vi "Write ITX (XY).vi"(4 "Commands":string, 6 "Notes":string, 8 "error in":errorcluster, 9 "wavenames":string[](array[string]), 10 "XY Array":cluster{"X  array":dbl[], "Y  Array":dbl[]}[](array[cluster]), 11 "filename":path) -> (0 "error out":errorcluster, 3 "file":path)   [LabVIEW 2016, in "Data.ITX.lvclass"]
uses:
  Data.ITX.lvclass
panel:
  out "String":string
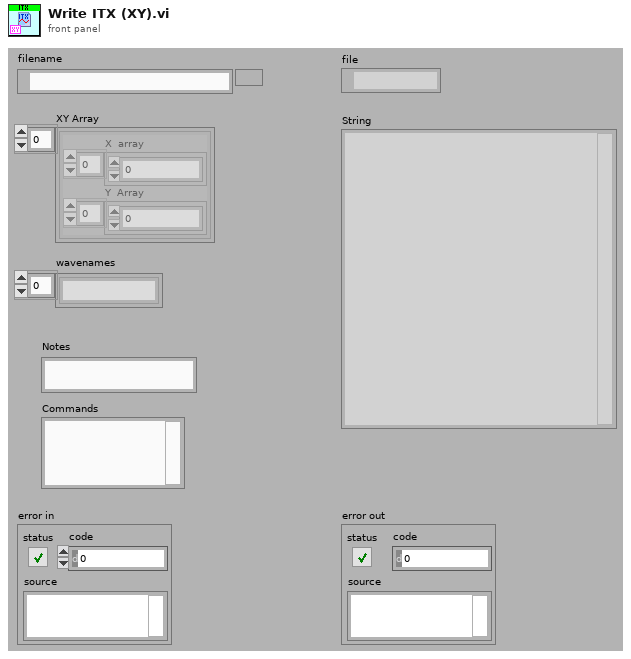
[diagram p1: front panel]
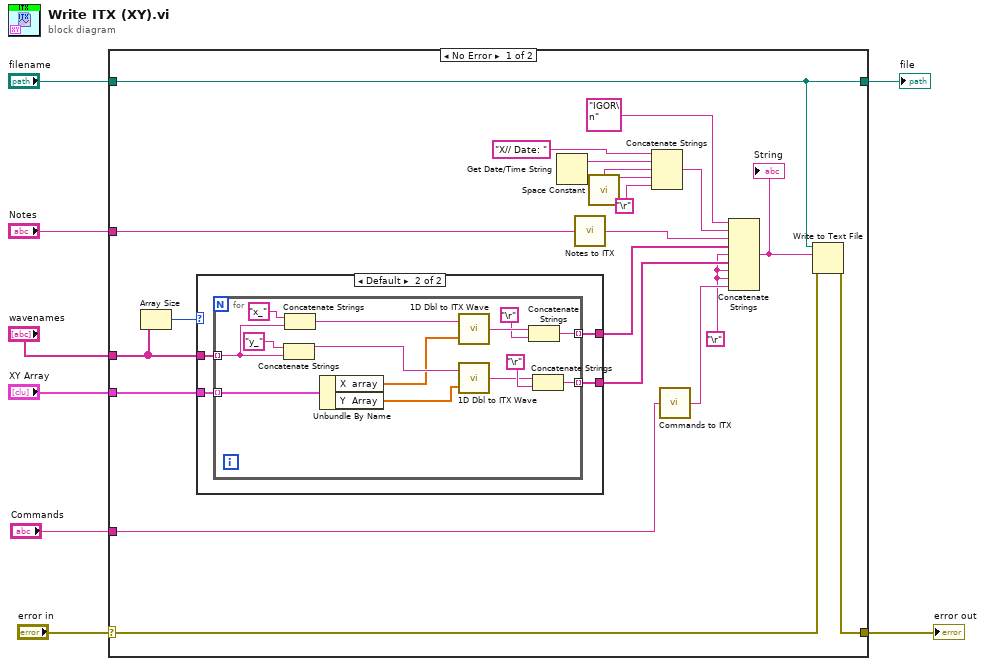
[diagram p0: block diagram]
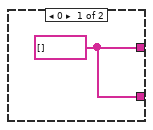
[diagram p2: hidden frame]
diagram:
  n1 = case shown="No Error" "error in" {
    selector: "error in" -> [w12 w50]
    tunnel: "filename" -> [w13 w49]
    tunnel: "wavenames" -> [w22 _]
    tunnel: "Notes" -> [w20 _]
    tunnel: "XY Array" -> [w19 _]
    tunnel: [w14 w50] -> w4
    tunnel: [w13 w49] -> w2
    tunnel: "Commands" -> [w10 _]
    frame No Error {
      w9 = "\r"
      n2 = Array Size(array=w22) -> (size(s)=w21:i32)
      n3 = case shown="Default" w21 {
        tunnel: w22 -> [_ w34]
        tunnel: w19 -> [_ w33]
        tunnel: [w30 w32] -> w24
        tunnel: [w30 w31] -> w11
        frame 0 {
          w30 = string[] []
        }
        frame Default {
          n4 = for {
            tunnel: [w48] -> w32 mode=indexing
            tunnel: w34 -> [w39] mode=indexing
            tunnel: w33 -> [w40] mode=indexing
            tunnel: [w43] -> w31 mode=indexing
            n5 = Concatenate Strings("y_" ("string"), w39) -> (w37:string)
            n6 = Concatenate Strings("x_" ("string"), w39) -> (w38:string)
            n7 = Unbundle By Name(w40) -> ("X  array"=w36:dbl[], "Y  Array"=w35:dbl[])
            n8 = call "1D Dbl to ITX Wave.vi"("1D Array"=w36, "Wavename"=w38) -> ("ITX Wave"=w47:string)
            n9 = call "1D Dbl to ITX Wave.vi"("1D Array"=w35, "Wavename"=w37) -> ("ITX Wave"=w44:string)
            n10 = Concatenate Strings(w47, "\r") -> (w48:string)
            n11 = Concatenate Strings(w44, "\r") -> (w43:string)
          }
        }
      }
      n12 = Get Date/Time String() -> (date string=w28:string, time string=w29:string)  [unwired: 3 out]
      n13 = call "Notes to ITX.vi"("Notes"=w20) -> ("ITX Notes"=w15:string)
      n14 = call <vilib>:"Space Constant.vi"() -> ("String"=w26:string)
      n15 = Concatenate Strings("X// Date: " ("format string"), w28, w26, w29, "\r") -> (w17:string)
      n16 = call "Commands to ITX.vi"("Commands"=w10) -> ("ITX Commands"=w18:string)
      n17 = Concatenate Strings("IGOR\n", w17, w15, w24, w9, w11, w9, w9, w18) -> (w23:string)
      "String" <- w23
      n18 = Write to Text File(file (use dialog)=w13, text=w23, error in=w12) -> (error out=w14:errorcluster)  [unwired: 3 out]
    }
    frame Error {
    }
  }
  "file" <- w2
  "error out" <- w4
